vi "String, Size to Text.vi"(8 "error in":errorcluster, 10 "string ref":refnum<vi>) -> (0 "error out":errorcluster, 2 "string ref dup":refnum<vi>)   [LabVIEW 2010]
doc: "This function performs a \"Size to Text\" operation on a string control.\n\nIn LabVIEW 2011 the \"Size to Text\" method does not properly size a multiline string."
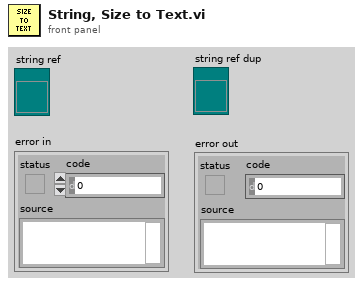
[diagram p1: front panel]
types:
  T1 = cluster{"Font Name:":string, "Size":i16, "Strikeout?":bool, "Italic?":bool, "Underline?":bool, "Outline?":bool, "Shadow?":bool, "Bold?":bool}
  T2 = enum16{"User-specified Font", "Application Font", "System Font", "Dialog Font"}
  T3 = typedef "LVFontTypeDef.ctl" = cluster{"Font Name":string, "Size":u16, "Bold":bool, "Italic":bool, "Underline":bool, "Strikeout":bool, "Color":u32}
  T4 = cluster{"left":i16, "top":i16, "right":i16, "bottom":i16}
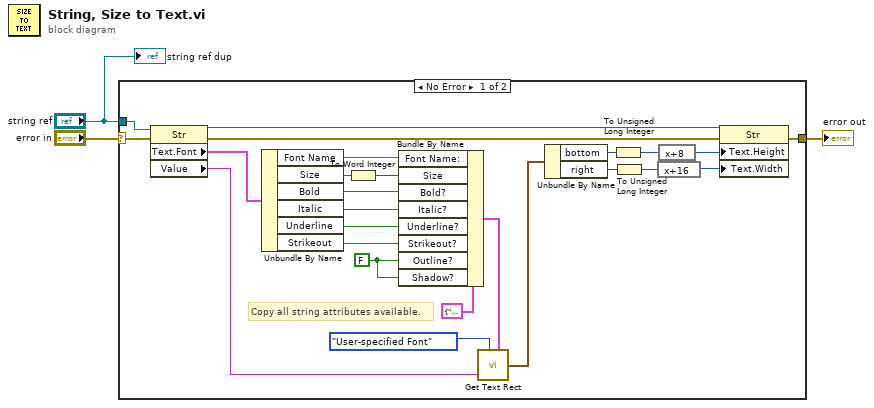
[diagram p0: block diagram]
diagram:
  n1 = case shown="No Error" "error in" {
    selector: "error in" -> [w4 w29]
    tunnel: [w28 w29] -> w3
    tunnel: "string ref" -> [w10 _]
    frame No Error {
      w5 = FALSE ("Outline?")
      # "Copy all string attributes available."
      n2 = property class="Str"(reference=w10, error in=w4) -> (reference out=w26:refnum<vi>, error out=w9:errorcluster, "Text.Font"=w8:T3, "Value"=w25:string)
      n3 = Unbundle By Name(w8) -> ("Font Name"=w24:string, "Size"=w12:u16, "Bold"=w22:bool, "Italic"=w15:bool, "Underline"=w14:bool, "Strikeout"=w13:bool)
      n4 = To Word Integer(number=w12) -> (16bit integer=w11:i16)
      n5 = Bundle By Name(cluster=T1 {"Font Name:"="", "Size"=0, "Strikeout?"=FALSE, "Italic?"=FALSE, "Underline?"=FALSE, "Outline?"=FALSE, "Shadow?"=FALSE, "Bold?"=FALSE} ("[user-specified font]"), "Font Name:"=w24, "Size"=w11, "Bold?"=w22, "Italic?"=w15, "Underline?"=w14, "Strikeout?"=w13, "Outline?"=w5, "Shadow?"=w5) -> (w23:T1)
      n6 = call <vilib>:"Get Text Rect.vi"("desired font(Application)"=T2."User-specified Font", "text"=w25, "[user-specified font]"=w23) -> ("rect"=w27:T4)  [unwired: 6 in]
      n7 = Unbundle By Name(w27) -> ("bottom"=w16:i16, "right"=w20:i16)
      n8 = To Unsigned Long Integer(number=w16) -> (unsigned 32bit integer=w17:u32)
      n9 = To Unsigned Long Integer(number=w20) -> (unsigned 32bit integer=w19:u32)
      n10 = expression code="x+16"(w19) -> (w18:u32)
      n11 = expression code="x+8"(w17) -> (w21:u32)
      n12 = property class="Str"(reference=w26, error in=w9, "Text.Height"=w21, "Text.Width"=w18) -> (error out=w28:errorcluster)  [unwired: 1 out]
    }
    frame Error {
    }
  }
  "error out" <- w3
  "string ref dup" <- "string ref"
